vi "Table_ColumnValue_Tests.vi"(8 "error in":errorcluster) -> (0 "error out":errorcluster)   [LabVIEW 2016, in "DronaTest.lvlib"]
uses:
  DronaTest.lvlib
  APIs/Stimulus/ControlValue/SetValueAuto.vi
  APIs/Stimulus/ControlValue/Controls/Table/EditColumnValue.vi
  APIs/Assert/AssertControlValue/Controls/Table/AssertColumnValue.vi
  <vilib>/addons/_JKI Toolkits/Caraya/classes/Assert/Assert Error.vi
  APIs/Stimulus/ControlValue/Controls/Table/SetValue.vi
  <vilib>/addons/_JKI Toolkits/Caraya/classes/Test/Test.lvclass
  <vilib>/SLL Toolkit/SLL Debug/SLL Debug.lvlib
  Drona.lvlib
  <vilib>/addons/_JKI Toolkits/Caraya/classes/Assert/Assert.lvclass
  APIs/Stimulus/ControlValue/ControlValue.lvlib
  APIs/Stimulus/ControlValue/Controls/Table/StimulusTable.lvlib
  APIs/Assert/AssertControlValue/Controls/Table/AssertTable.lvlib
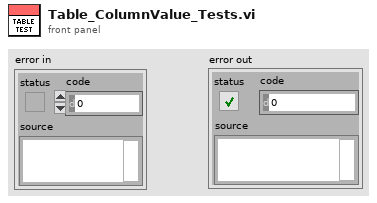
[diagram p1: front panel]
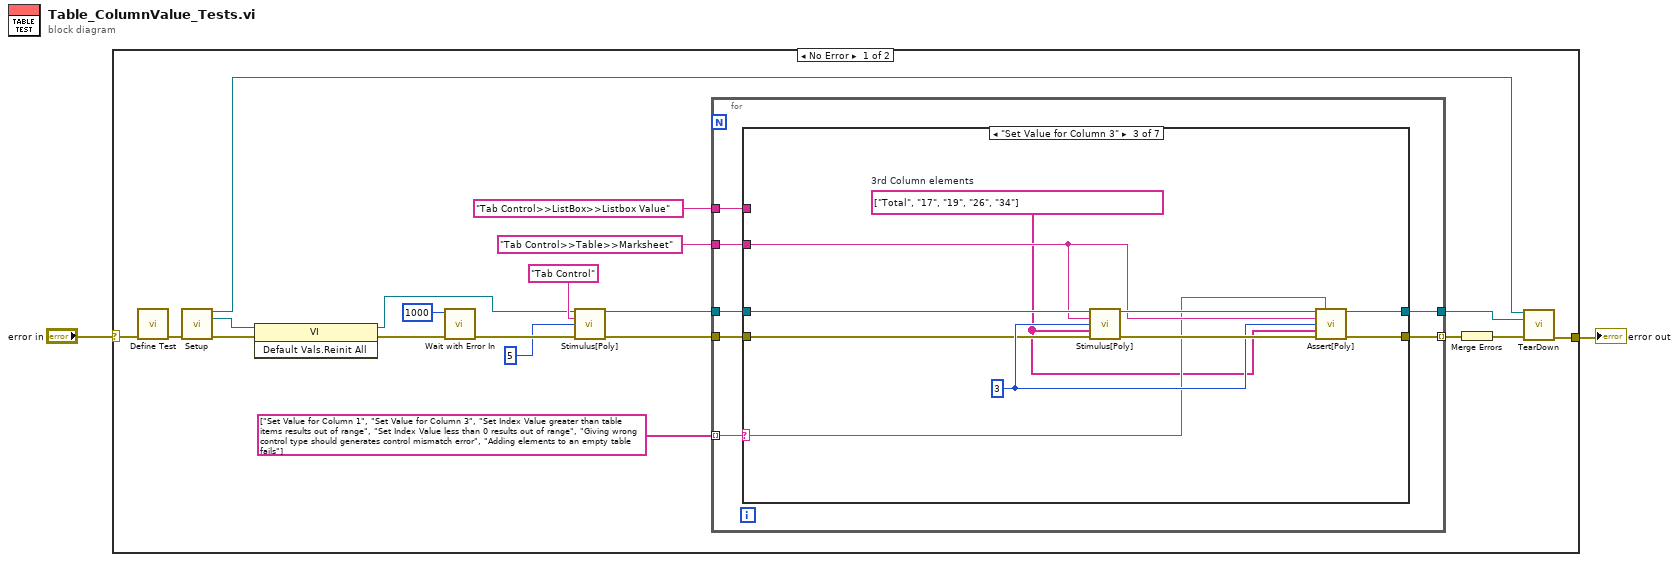
[diagram p0: block diagram]
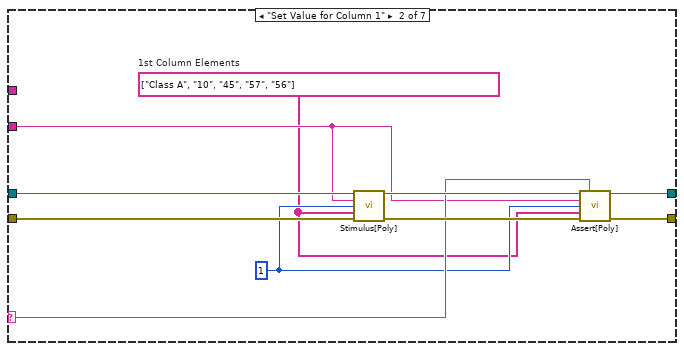
[diagram p3: hidden frame]
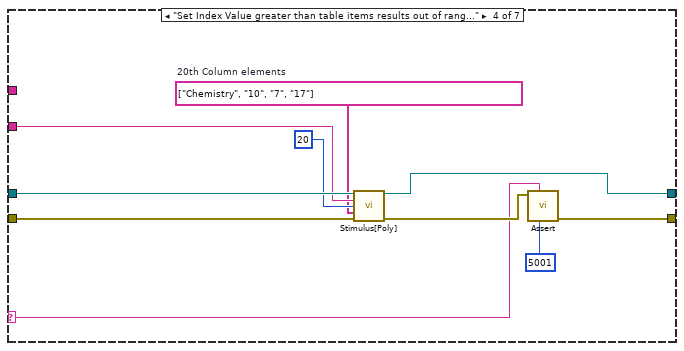
[diagram p4: hidden frame]
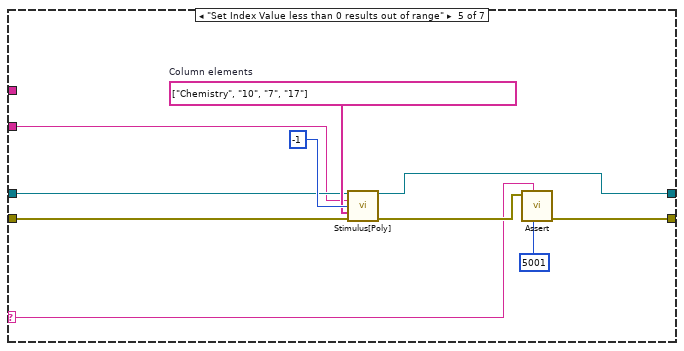
[diagram p5: hidden frame]
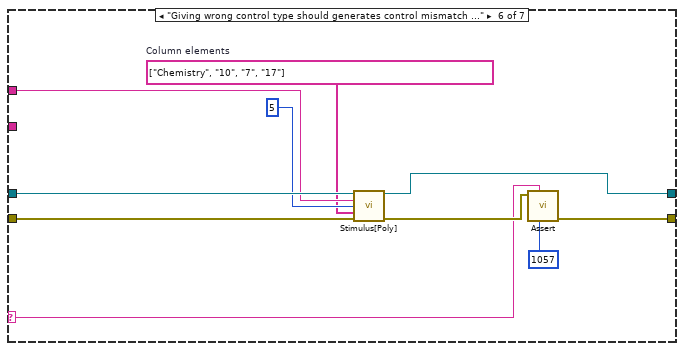
[diagram p6: hidden frame]
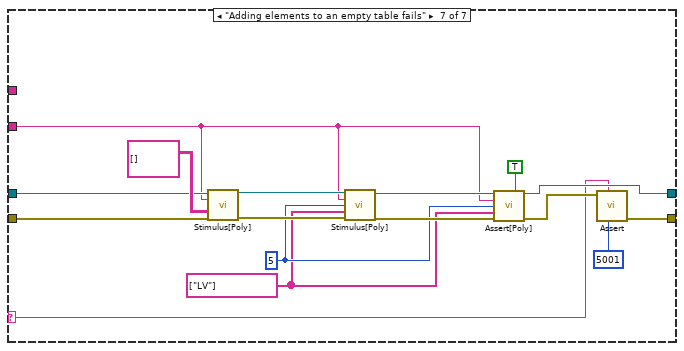
[diagram p7: hidden frame]
diagram:
  n1 = case shown="No Error" "error in" {
    selector: "error in" -> [w22 w98]
    tunnel: [w7 w98] -> w1
    frame No Error {
      n2 = call <vilib>:"Define Test.vi"("error in (no error)"=w22) -> ("error out"=w12:errorcluster)  [unwired: 9 in, 1 out]
      n3 = call "Setup.vi"("error in"=w12) -> ("Application Ref"=w9:refnum<vi>, "VI out"=w4:refnum<vi>, "error out"=w11:errorcluster)  [unwired: 12 in]
      n4 = invoke class="VI" method="Default Vals.Reinit All"(reference=w4, error in=w11) -> (reference out=w3:refnum<vi>, error out=w5:errorcluster)  [unwired: 1 in, 1 out]
      n5 = call <vilib>:"Wait with Error In.vi"("error in (no error)"=w5, "milliseconds to wait"=u32 1000) -> ("error out"=w20:errorcluster)  [unwired: 9 in]
      n6 = call-poly "Stimulus[Poly].vi"("VI Reference In"=w3, "Control Path"="Tab Control", "Value (Signaling)"=5, "error in"=w20) -> ("VI Reference Out"=w16:refnum<vi>, "error out"=w19:errorcluster)  [unwired: 10 in]
      n7 = for {
        tunnel: w16 -> [w28]
        tunnel: "Tab Control>>Table>>Marksheet" ("Control Path") -> [w27]
        tunnel: "Tab Control>>ListBox>>Listbox Value" ("Control Path") -> [w26]
        tunnel: string[] ["Set Value for Column 1", "Set Value for Column 3", "Set Index Value greater than table items results out of range", "Set Index Value less than 0 results out of range", "Giving wrong control type should generates control mismatch error", "Adding elements to an empty table fails"] -> [w24] mode=indexing
        tunnel: [w23] -> w8
        tunnel: w19 -> [w29]
        tunnel: [w25] -> w13 mode=indexing
        n8 = case shown="\"Set Value for Column 3\"" w24 {
          selector: w24 -> [_ w35 w43 w56 w63 w77 w82]
          tunnel: w29 -> [w31 w41 w48 w61 w66 w81 w87]
          tunnel: w28 -> [w30 w40 w47 w60 w67 w80 w86]
          tunnel: w27 -> [_ w34 w46 w59 w62 _ w85]
          tunnel: w26 -> [_ _ _ _ _ w74 _]
          tunnel: [w31 w37 w44 w57 w65 w78 w84] -> w25
          tunnel: [w30 w36 w45 w54 w64 w75 w83] -> w23
          frame Default {
          }
          frame "Set Value for Column 1" {
            w32 = string[] ["Class A", "10", "45", "57", "56"]  # 1st Column Elements
            w33 = 1 ("Item Index")
            n9 = call-poly "Stimulus[Poly].vi"("VI Reference In"=w40, "Control Path"=w34, "Column Index"=w33, "Value"=w32, "Error In"=w41) -> ("VI Reference Out"=w38:refnum<vi>, "Error Out"=w39:errorcluster)  [unwired: 9 in]
            n10 = call-poly "Assert[Poly].vi"("VI Reference In"=w38, "Test Label"=w35, "Control Path"=w34, "Column Index"=w33, "Item Value"=w32, "Error In"=w39) -> ("VI Reference Out"=w36:refnum<vi>, "Error Out"=w37:errorcluster)  [unwired: 7 in, 1 out]
          }
          frame "Set Value for Column 3" {
            w42 = string[] ["Total", "17", "19", "26", "34"]  # 3rd Column elements
            w49 = 3 ("Item Index")
            n11 = call-poly "Stimulus[Poly].vi"("VI Reference In"=w47, "Control Path"=w46, "Column Index"=w49, "Value"=w42, "Error In"=w48) -> ("VI Reference Out"=w50:refnum<vi>, "Error Out"=w51:errorcluster)  [unwired: 9 in]
            n12 = call-poly "Assert[Poly].vi"("VI Reference In"=w50, "Test Label"=w43, "Control Path"=w46, "Column Index"=w49, "Item Value"=w42, "Error In"=w51) -> ("VI Reference Out"=w45:refnum<vi>, "Error Out"=w44:errorcluster)  [unwired: 7 in, 1 out]
          }
          frame "Set Index Value greater than table items results out of range" {
            w52 = string[] ["Chemistry", "10", "7", "17"]  # 20th Column elements
            n13 = call-poly "Stimulus[Poly].vi"("VI Reference In"=w60, "Control Path"=w59, "Column Index"=20 ("Item Index"), "Value"=w52, "Error In"=w61) -> ("VI Reference Out"=w54:refnum<vi>, "Error Out"=w58:errorcluster)  [unwired: 9 in]
            n14 = call-poly <vilib>:"Assert.vi"("error code (1)"=5001, "Label"=w56, "Error?"=w58) -> ("error out"=w57:errorcluster)  [unwired: 7 in, 1 out]
          }
          frame "Set Index Value less than 0 results out of range" {
            w68 = string[] ["Chemistry", "10", "7", "17"]  # Column elements
            n15 = call-poly "Stimulus[Poly].vi"("VI Reference In"=w67, "Control Path"=w62, "Column Index"=-1 ("Item Index"), "Value"=w68, "Error In"=w66) -> ("VI Reference Out"=w64:refnum<vi>, "Error Out"=w71:errorcluster)  [unwired: 9 in]
            n16 = call-poly <vilib>:"Assert.vi"("error code (1)"=5001, "Label"=w63, "Error?"=w71) -> ("error out"=w65:errorcluster)  [unwired: 7 in, 1 out]
          }
          frame "Giving wrong control type should generates control mismatch error" {
            w72 = string[] ["Chemistry", "10", "7", "17"]  # Column elements
            n17 = call-poly "Stimulus[Poly].vi"("VI Reference In"=w80, "Control Path"=w74, "Column Index"=5 ("Item Index"), "Value"=w72, "Error In"=w81) -> ("VI Reference Out"=w75:refnum<vi>, "Error Out"=w79:errorcluster)  [unwired: 9 in]
            n18 = call-poly <vilib>:"Assert.vi"("error code (1)"=1057, "Label"=w77, "Error?"=w79) -> ("error out"=w78:errorcluster)  [unwired: 7 in, 1 out]
          }
          frame "Adding elements to an empty table fails" {
            w88 = string[] ["LV"] ("Value")
            w89 = 5 ("Row Index")
            n19 = call-poly "Stimulus[Poly].vi"("VI Reference In"=w86, "Control Path"=w85, "Value"=string[][] [], "Error In"=w87) -> ("VI Reference Out"=w95:refnum<vi>, "Error Out"=w97:errorcluster)  [unwired: 10 in]
            n20 = call-poly "Stimulus[Poly].vi"("VI Reference In"=w95, "Control Path"=w85, "Column Index"=w89, "Value"=w88, "Error In"=w97) -> ("VI Reference Out"=w93:refnum<vi>, "Error Out"=w94:errorcluster)  [unwired: 9 in]
            n21 = call-poly "Assert[Poly].vi"("VI Reference In"=w93, "Assert Only? (F)"=TRUE, "Control Path"=w85, "Column Index"=w89, "Item Value"=w88, "Error In"=w94) -> ("VI Reference Out"=w83:refnum<vi>, "Error Out"=w91:errorcluster)  [unwired: 7 in, 1 out]
            n22 = call-poly <vilib>:"Assert.vi"("error code (1)"=5001, "Label"=w82, "Error?"=w91) -> ("error out"=w84:errorcluster)  [unwired: 7 in, 1 out]
          }
        }
      }
      n23 = Merge Errors(w13) -> (w10:errorcluster)
      n24 = call "TearDown.vi"("Application Ref"=w9, "VI in"=w8, "error in (no error)"=w10) -> ("error out"=w7:errorcluster)  [unwired: 12 in]
    }
    frame Error {
    }
  }
  "error out" <- w1
